vi "Write MXN.vi"(8 "error in (no error)":errorcluster, 10 "MXN":bool, 11 "Actor M in":refnum<class "Actor M.lvclass">) -> (0 "error out":errorcluster, 3 "Actor M out":refnum<class "Actor M.lvclass">)   [LabVIEW 2019, in "Actor M.lvlib" / "Actor M.lvclass"]
uses:
  Actor M.lvclass
  Actor M.lvclass/Actor M.ctl
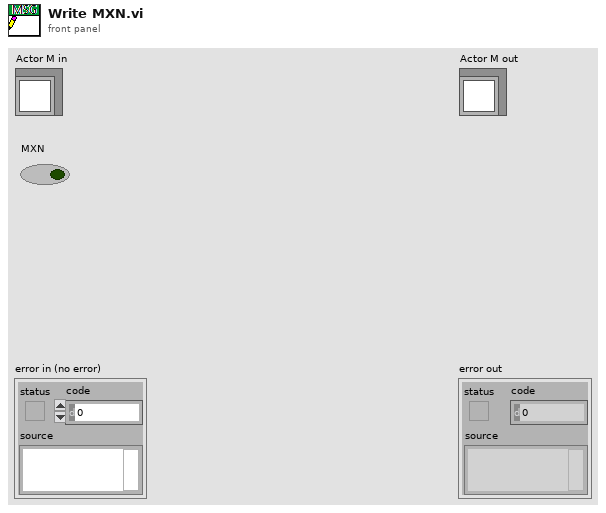
[diagram p1: front panel]
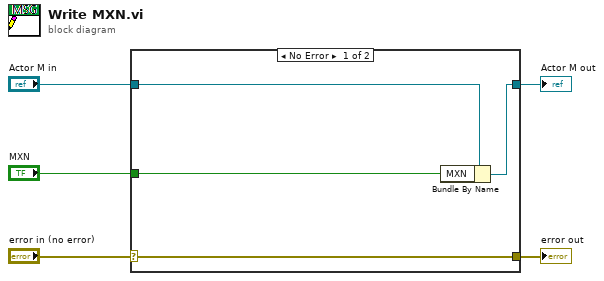
[diagram p0: block diagram]
diagram:
  n1 = case shown="No Error" "error in (no error)" {
    selector: "error in (no error)" -> [w9 w10]
    tunnel: [w9 w10] -> w4
    tunnel: [w7 w11] -> w2
    tunnel: "Actor M in" -> [w8 w11]
    tunnel: "MXN" -> [w6 _]
    frame No Error {
      n2 = Bundle By Name(cluster=w8, "MXN"=w6) -> (w7:refnum<class "Actor M.lvclass">)
    }
    frame Error {
    }
  }
  "error out" <- w4
  "Actor M out" <- w2
